vi "ThorlabsOCT Module.vi"() -> ()   [LabVIEW 2014]
uses:
  user.lib/SpectralRadar.llb/OCT Device.lvclass
  user.lib/SpectralRadar.llb/Processing.lvclass
  user.lib/SpectralRadar.llb/Probe.lvclass
  Controls/ThorlabsOCT Module Contols.ctl
  user.lib/SpectralRadar.llb/Raw Data.lvclass
  user.lib/SpectralRadar.llb/Scan Pattern.lvclass
  Controls/ThorlabsOCT Scan Parameters.ctl
  user.lib/SpectralRadar.llb/Processing Parameter Int Selection.ctl
  user.lib/SpectralRadar.llb/Probe Parameter Int Selection.ctl
panel:
  in  "BScan angle \n[deg]":dbl(knob) scale=0.0..180.0 scale format="%#.6g"
  in  "BScan\nY offset [mm]":dbl min=-5.0 max=5.0 format="%_4f"
  in  "BScan\nX offset [mm]":dbl min=-5.0 max=5.0 format="%_4f"
  in  "Thorlabs OCT Scan Parameters":T1={"Index of Refraction"=1.0, "Columns"=1000, "Range X [mm]"=2.0, "B-Scan Averaging"=1, "BScan X offset [mm]"=0.0, "BScan Y offset [mm]"=0.0, "BScan angle [deg]"=0.0, "Window"=enum."Hann", "Spectral Ave."=0, "A-Scan Ave."=0} {"BScan Y offset [mm]" min=-5.0 max=5.0 format="%_4f"; "BScan X offset [mm]" min=-5.0 max=5.0 format="%_4f"; "B-Scan Averaging" min=1 max=20 step=1; "Range X [mm]" min=0.0 max=10.0 step=0.5 format="%_3f"; "Columns" min=50 max=10240 step=1; "Index of Refraction" min=1.0 max=5.0 step=0.10000000149011612 format="%.3f"}
  in  "Action":T2=enum."Uninit"
  out "Error Out":errorcluster
  in  "Error In":errorcluster
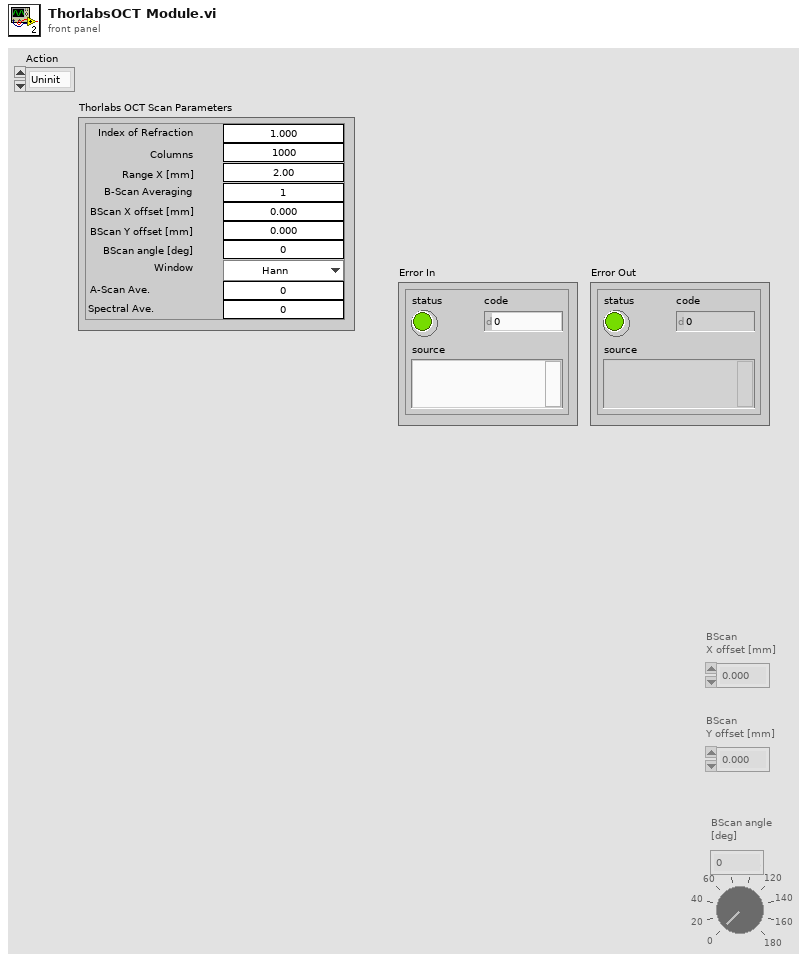
[diagram p1: front panel]
types:
  T1 = typedef "ThorlabsOCT Scan Parameters.ctl" = cluster{"Index of Refraction":dbl, "Columns":i32, "Range X [mm]":dbl, "B-Scan Averaging":i32, "BScan X offset [mm]":dbl, "BScan Y offset [mm]":dbl, "BScan angle [deg]":dbl, "Window":enum16{"Hann", "Hamming", "Gauss", "Tapered Cosine", "Blackman", "4 Term B-Harris"}, "Spectral Ave.":i32, "A-Scan Ave.":i32}
  T2 = typedef "ThorlabsOCT Module Contols.ctl" = enum16{"Init", "Configure Scan", "Start Scan", "Configure FOV", "Configure Averaging", "End Scan", "Uninit"}
  T3 = typedef "Probe.lvclass/Probe Parameter Int Selection.ctl" = enum16{"Apodization Cycles", "Oversampling", "Oversampling Slow Axis", "Speckle Reduction"}
  T4 = typedef "Processing.lvclass/Processing Parameter Int Selection.ctl" = enum32{"Spectrum Averaging", "A-Scan Averaging", "B-Scan Averaging", "Zero Padding", "Number of Threads", "Fourier Averaging"}
  T5 = enum16{"Asynchronous Continuous", "Asynchronous Finite", "Synchronous"}
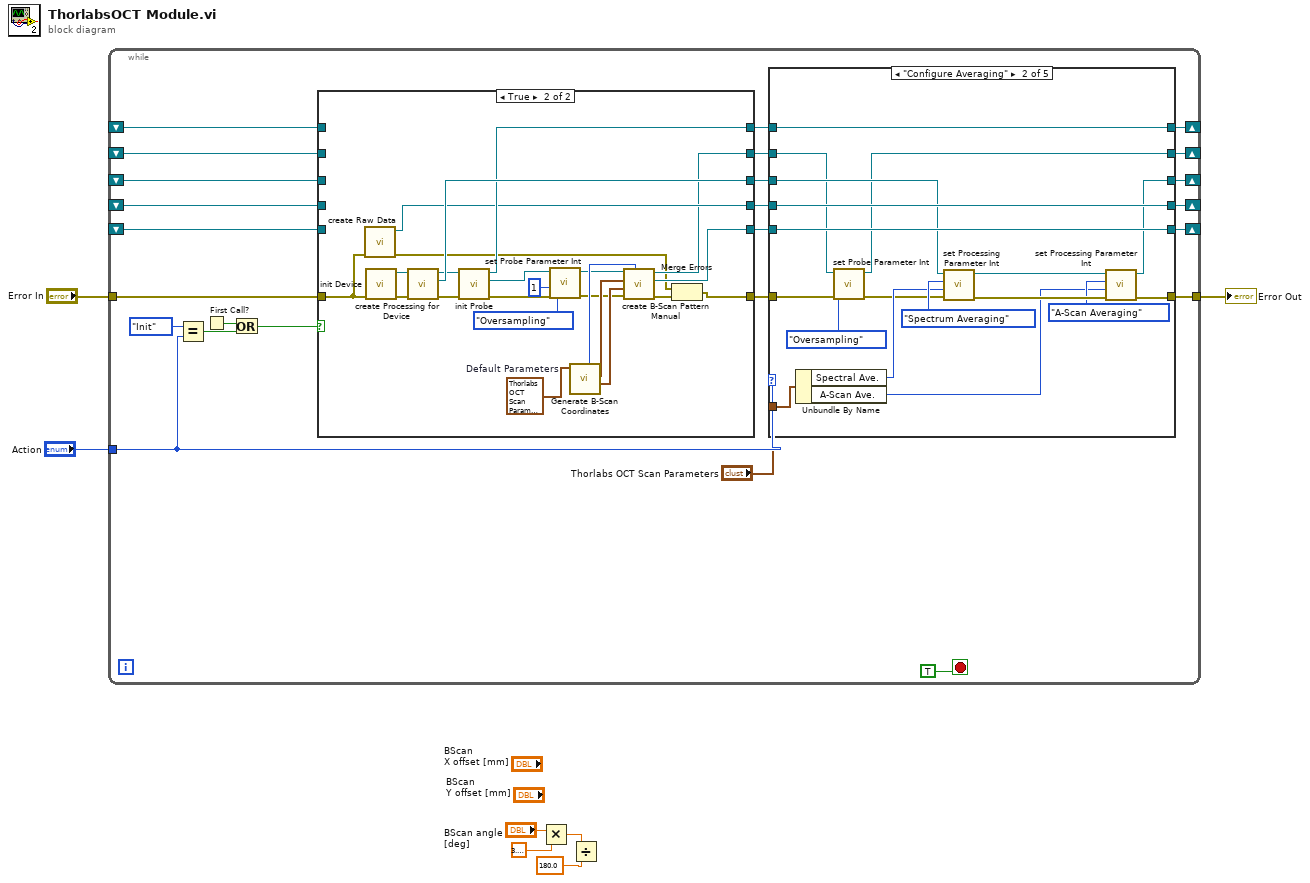
[diagram p0: block diagram]
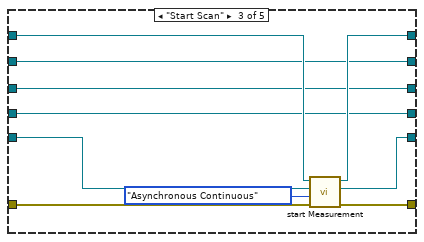
[diagram p3: hidden frame]
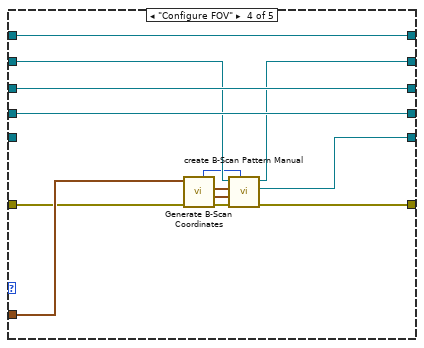
[diagram p4: hidden frame]
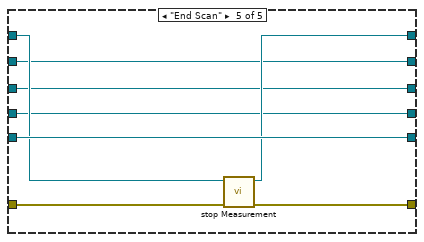
[diagram p5: hidden frame]
diagram:
  n1 = while {
    tunnel: "Action" -> [w17]
    tunnel: "Error In" -> [w31]
    tunnel: [w12] -> w5
    shift-right: [w18] -> _
    shift-left: _ -> [w30]
    shift-right: [w20] -> _
    shift-left: _ -> [w29]
    shift-right: [w19] -> _
    shift-left: _ -> [w28]
    shift-right: [w15] -> _
    shift-left: _ -> [w14]
    shift-right: [w10] -> _
    shift-left: _ -> [w9]
    stop <- TRUE stop-if-true
    n2 = Equal?(x=ThorlabsOCT_Module_Contols."Init", y=w17) -> (x = y?=w26:bool)
    n3 = First Call?() -> (First Call?: T/F=w25:bool)
    n4 = Or(x=w25, y=w26) -> (x .or. y?=w24:bool)
    n5 = case shown="True" w24 {
      tunnel: w31 -> [w89 w107]
      tunnel: [w91 w111] -> w21
      tunnel: w30 -> [w91 _]
      tunnel: [w93 w114] -> w23
      tunnel: w29 -> [w93 _]
      tunnel: [w92 w108] -> w22
      tunnel: w28 -> [w92 _]
      tunnel: [w89 w103] -> w13
      tunnel: [w90 w110] -> w16
      tunnel: w14 -> [w90 _]
      tunnel: [w88 w109] -> w11
      tunnel: w9 -> [w88 _]
      frame False {
      }
      frame True {
        w106 = T1 {"Index of Refraction"=1.0, "Columns"=1000, "Range X [mm]"=2.0, "B-Scan Averaging"=1, "BScan X offset [mm]"=0.0, "BScan Y offset [mm]"=0.0, "BScan angle [deg]"=0.0, "Window"=enum."Hann", "Spectral Ave."=0, "A-Scan Ave."=0}  # Default Parameters
        n6 = call "create Raw Data.vi"("error in (no error)"=w107) -> ("error out"=w102:errorcluster, "Raw Data"=w110:refnum<class "Raw Data.lvclass">)  [unwired: 5 in]
        n7 = call "init Device.vi"("error in (no error)"=w107) -> ("error out"=w116:errorcluster, "OCTDevice"=w115:refnum<class "OCT Device.lvclass">)  [unwired: 5 in]
        n8 = call "create Processing for Device.vi"("error in (no error)"=w116, "OCTDevice"=w115) -> ("error out"=w113:errorcluster, "Processing"=w114:refnum<class "Processing.lvclass">, "OCTDevice"=w112:refnum<class "OCT Device.lvclass">)  [unwired: 3 in]
        n9 = call "init Probe.vi"("error in (no error)"=w113, "OCT Device [In]"=w112) -> ("error out"=w100:errorcluster, "GalvoControl"=w96:refnum<class "Probe.lvclass">, "OCT Device [Out]"=w111:refnum<class "OCT Device.lvclass">)  [unwired: 3 in]
        n10 = call "set Probe Parameter Int.vi"("error in (no error)"=w100, "Value"=1, "Probe Parameter Int"=Probe_Parameter_Int_Selection."Oversampling", "GalvoControl"=w96) -> ("error out"=w99:errorcluster, "GalvoControl"=w97:refnum<class "Probe.lvclass">)  [unwired: 2 in]
        n11 = call "Generate B-Scan Coordinates.vi"("Thorlabs OCT Scan Parameters [in]"=w106) -> ("End Coordinates"=w104:cluster{"Start X":dbl, "Start Y":dbl}, "Start Coordinates"=w105:cluster{"Start X":dbl, "Start Y":dbl}, "Num A-Lines"=w101:i32)  [unwired: 6 in, 2 out]
        n12 = call "create B-Scan Pattern Manual.vi"("AScans"=w101, "error in (no error)"=w99, "Stop"=w104, "Start"=w105, "Probe in"=w97) -> ("error out"=w98:errorcluster, "Scan Pattern"=w109:refnum<class "Scan Pattern.lvclass">, "Probe out"=w108:refnum<class "Probe.lvclass">)  [unwired: 2 in]
        n13 = Merge Errors(w102, w98) -> (w103:errorcluster)
      }
    }
    n14 = case shown="\"Configure Averaging\"" w17 {
      tunnel: w23 -> [w38 w48 w58 w78 w81]
      tunnel: w22 -> [w37 w41 w59 w70 w80]
      tunnel: w21 -> [w36 w56 w64 w79 w84]
      tunnel: [w38 w47 w58 w78 w81] -> w20
      tunnel: [w37 w40 w59 w69 w80] -> w19
      tunnel: [w36 w56 w63 w79 w83] -> w18
      tunnel: w16 -> [w35 w55 w57 w77 w82]
      tunnel: [w35 w55 w57 w77 w82] -> w15
      tunnel: w13 -> [w33 w43 w66 w71 w87]
      tunnel: [w33 w49 w65 w74 w86] -> w12
      tunnel: w11 -> [w34 w54 w62 _ w85]
      tunnel: [w34 w54 w61 w68 w85] -> w10
      tunnel: "Thorlabs OCT Scan Parameters" -> [_ w46 _ w75 _]
      frame "Init" {
      }
      frame "Configure Averaging" {
        n15 = Unbundle By Name(w46) -> ("Spectral Ave."=w45:i32, "A-Scan Ave."=w44:i32)
        n16 = call "set Probe Parameter Int.vi"("error in (no error)"=w43, "Probe Parameter Int"=Probe_Parameter_Int_Selection."Oversampling", "GalvoControl"=w41) -> ("error out"=w42:errorcluster, "GalvoControl"=w40:refnum<class "Probe.lvclass">)  [unwired: 3 in]
        n17 = call "set Processing Parameter Int.vi"("error in (no error)"=w42, "Value"=w45, "Processing Paramter Int Selection"=Processing_Parameter_Int_Selection."Spectrum Averaging", "Processing in"=w48) -> ("error out"=w51:errorcluster, "Processing out"=w52:refnum<class "Processing.lvclass">)  [unwired: 2 in]
        n18 = call "set Processing Parameter Int.vi"("error in (no error)"=w51, "Value"=w44, "Processing Paramter Int Selection"=Processing_Parameter_Int_Selection."A-Scan Averaging", "Processing in"=w52) -> ("error out"=w49:errorcluster, "Processing out"=w47:refnum<class "Processing.lvclass">)  [unwired: 2 in]
      }
      frame "Start Scan" {
        n19 = call "start Measurement.vi"("error in (no error)"=w66, "Acquisition Type"=T5."Asynchronous Continuous", "Scan Pattern"=w62, "OCTDevice"=w64) -> ("error out"=w65:errorcluster, "Scan Pattern"=w61:refnum<class "Scan Pattern.lvclass">, "OCTDevice"=w63:refnum<class "OCT Device.lvclass">)  [unwired: 1 in]
      }
      frame "Configure FOV" {
        n20 = call "Generate B-Scan Coordinates.vi"("Error In"=w71, "Thorlabs OCT Scan Parameters [in]"=w75) -> ("Error Out"=w72:errorcluster, "End Coordinates"=w76:cluster{"Start X":dbl, "Start Y":dbl}, "Start Coordinates"=w73:cluster{"Start X":dbl, "Start Y":dbl}, "Num A-Lines"=w67:i32)  [unwired: 5 in, 1 out]
        n21 = call "create B-Scan Pattern Manual.vi"("AScans"=w67, "error in (no error)"=w72, "Stop"=w76, "Start"=w73, "Probe in"=w70) -> ("error out"=w74:errorcluster, "Scan Pattern"=w68:refnum<class "Scan Pattern.lvclass">, "Probe out"=w69:refnum<class "Probe.lvclass">)  [unwired: 2 in]
      }
      frame "End Scan" {
        n22 = call "stop Measurement.vi"("error in (no error)"=w87, "OCTDevice"=w84) -> ("error out"=w86:errorcluster, "OCTDevice"=w83:refnum<class "OCT Device.lvclass">)  [unwired: 4 in]
      }
    }
  }
  "Error Out" <- w5
  n23 = Multiply(x="BScan angle \n[deg]", y=3.141592653589793) -> (x*y=w2:dbl)
  n24 = Divide(x=w2, y=180.0) -> ()  [unwired: 1 out]
